vi "ndipolaris Start Tracking.vi"(8 "error in (no error)":errorcluster, 9 "Reset Frame Counter? (F:No)":bool, 11 "VISA resource name":refnum<visa-resource-name>) -> (0 "error out":errorcluster, 3 "VISA resource out":refnum<visa-resource-name>)   [LabVIEW 2013]
doc: "This VI will put the instrument into tracking mode. The instrument can only return transformations when it is in tracking mode. The instrument will stay in tracking mode until the Stop Tracking VI has executed."
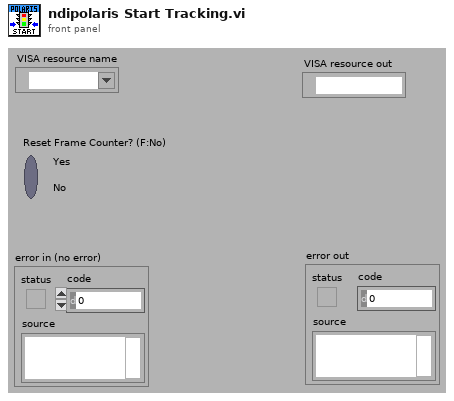
[diagram p1: front panel]
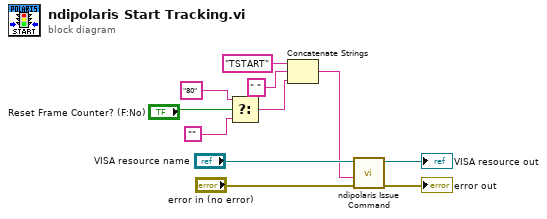
[diagram p0: block diagram]
diagram:
  n1 = Select(t="80" ("string"), s="Reset Frame Counter? (F:No)", f="") -> (s? t:f=w9:string)
  n2 = Concatenate Strings("TSTART" ("string"), " " ("string"), w9) -> (w5:string)
  n3 = call <instrlib>:"ndipolaris Issue Command.vi"("error in (no error)"="error in (no error)", "Write Buffer"=w5, "VISA resource name"="VISA resource name") -> ("error out"=→"error out":errorcluster, "VISA resource out"=→"VISA resource out":refnum<visa-resource-name>)  [unwired: 6 in, 1 out]
